vi "HEWH Draw Flag.vi"(0 "Station ID":T2, 1 "Status":T1, 11 "Error In":errorcluster) -> (4 "Station A":bool, 6 "Station B":bool, 8 "Station C":bool, 10 "Station D":bool, 15 "Error Out":errorcluster)   [LabVIEW 2016]
uses:
  Custom Instrument Control/MW100/Type Definitions/Station ID Selector.ctl
  Utility/Type Definitions/UTILITY Notifier.ctl
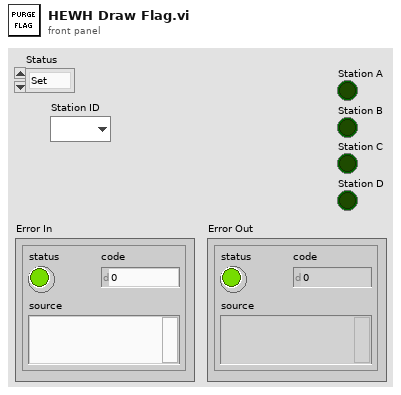
[diagram p1: front panel]
types:
  T1 = typedef "UTILITY Notifier.ctl" = enum16{"Set", "Read", "Release Ref"}
  T2 = typedef "Station ID Selector.ctl" = enum16{"", "A", "B", "C", "D", "Global"}
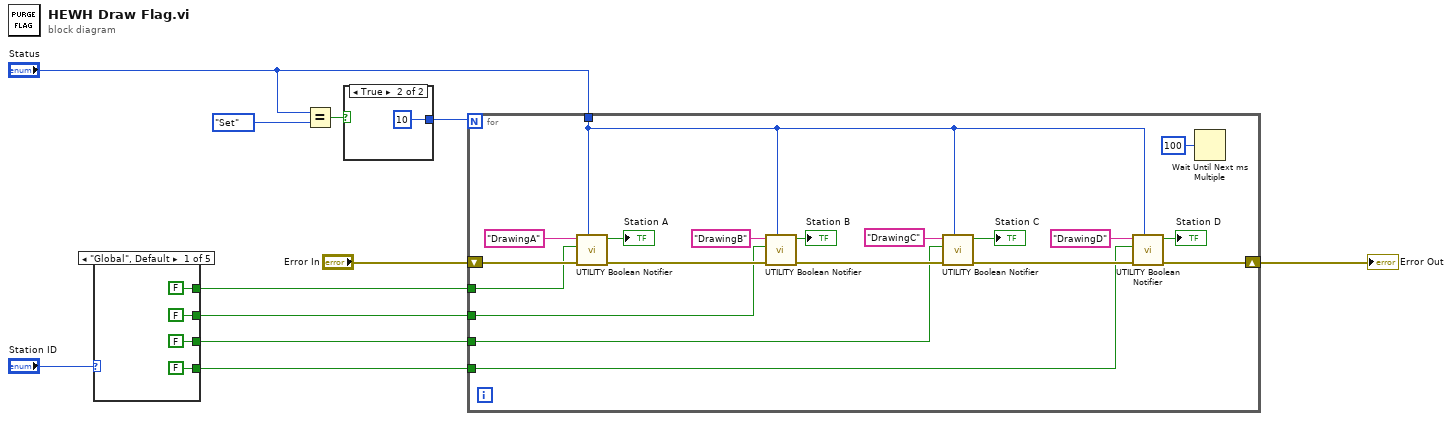
[diagram p0: block diagram]
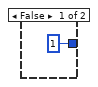
[diagram p2: hidden frame]
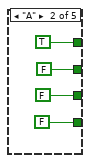
[diagram p3: hidden frame]
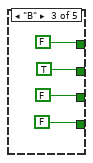
[diagram p4: hidden frame]
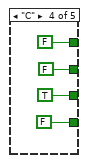
[diagram p5: hidden frame]
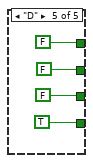
[diagram p6: hidden frame]
diagram:
  n1 = case shown="\"Global\", Default" "Station ID" {
    tunnel: [FALSE ("Set Status") TRUE ("Set Status") FALSE ("Set Status") FALSE ("Set Status") FALSE ("Set Status")] -> w9
    tunnel: [FALSE ("Set Status") FALSE ("Set Status") TRUE ("Set Status") FALSE ("Set Status") FALSE ("Set Status")] -> w8
    tunnel: [FALSE ("Set Status") FALSE ("Set Status") FALSE ("Set Status") TRUE ("Set Status") FALSE ("Set Status")] -> w7
    tunnel: [FALSE ("Set Status") FALSE ("Set Status") FALSE ("Set Status") FALSE ("Set Status") TRUE ("Set Status")] -> w6
    frame "Global", Default {
    }
    frame "A" {
    }
    frame "B" {
    }
    frame "C" {
    }
    frame "D" {
    }
  }
  n2 = Equal?(x="Status", y=UTILITY_Notifier."Set") -> (x = y?=w2:bool)
  n3 = case shown="True" w2 {
    tunnel: [1 10] -> w1
    frame False {
    }
    frame True {
    }
  }
  n4 = for {
    N: w1 -> [_]
    tunnel: w9 -> [w43]
    tunnel: w8 -> [w42]
    tunnel: w7 -> [w41]
    tunnel: w6 -> [w40]
    tunnel: "Status" -> [w35]
    shift-right: [w44] -> w10
    shift-left: "Error In" -> [w45]
    n5 = call "UTILITY Boolean Notifier.vi"("Status"=w35, "error in (no error)"=w45, "Set Status"=w43, "name (unnamed)"="DrawingA") -> ("error out"=w50:errorcluster, "latest READ notification"=→"Station A":bool)  [unwired: 6 in]
    n6 = call "UTILITY Boolean Notifier.vi"("Status"=w35, "error in (no error)"=w50, "Set Status"=w42, "name (unnamed)"="DrawingB") -> ("error out"=w51:errorcluster, "latest READ notification"=→"Station B":bool)  [unwired: 6 in]
    n7 = call "UTILITY Boolean Notifier.vi"("Status"=w35, "error in (no error)"=w51, "Set Status"=w41, "name (unnamed)"="DrawingC") -> ("error out"=w52:errorcluster, "latest READ notification"=→"Station C":bool)  [unwired: 6 in]
    n8 = call "UTILITY Boolean Notifier.vi"("Status"=w35, "error in (no error)"=w52, "Set Status"=w40, "name (unnamed)"="DrawingD") -> ("error out"=w44:errorcluster, "latest READ notification"=→"Station D":bool)  [unwired: 6 in]
    n9 = Wait Until Next ms Multiple(millisecond multiple=u32 100) -> ()  [unwired: 1 out]
  }
  "Error Out" <- w10
